vi "Write Base Actor DVR.vi"(10 "Base Actor DVR":refnum<data-value>, 11 "TEMPLATE Actor in":refnum<class "{{Name}}Actor.lvclass">) -> (3 "TEMPLATE Actor out":refnum<class "{{Name}}Actor.lvclass">)   [LabVIEW 2020, in "_Template.lvlib" / "Templates.lvlib" / "{{Name}}Actor.lvlib" / "{{Name}}Actor.lvclass"]
uses:
  {{Name}}Actor.lvclass
  {{Name}}Actor.lvclass/{{Name}}Actor.ctl
  jettl/jettl/ActorLifetime.ctl
  jettl/jettl/jettl.lvlib
  jettl/jettl/BaseActor.ctl
  jettl/jettl/Message/Message.lvclass
  jettl/jettl/MessageSet.ctl
  jettl/jettl/Messages.ctl
  jettl/jettl/Message.ctl
  jettl/jettl/ActorType.ctl
  jettl/jettl/Actor.ctl
  jettl/jettl/ActorMap.ctl
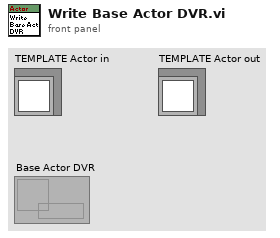
[diagram p1: front panel]
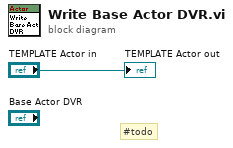
[diagram p0: block diagram]
diagram:
  # "#todo"
  "TEMPLATE Actor out" <- "TEMPLATE Actor in"
